vi "waveform temp.vi"() -> ()   [LabVIEW 2025]
panel:
  out "slide 2":u8(slide) scale=0.0..100.0
  out "slide 1":dbl(slide) scale=0.0..10.0
  out "iteration 2":dbl
  out "iteration 1":dbl
  out "Waveform Chart":dbl(graph)
  in  "mil per sec to wait":dbl
  in  "no of loops":dbl
  out "Waveform Graph":dbl[](graph)
  in  "mil per sec":dbl
  in  "no of loops":dbl
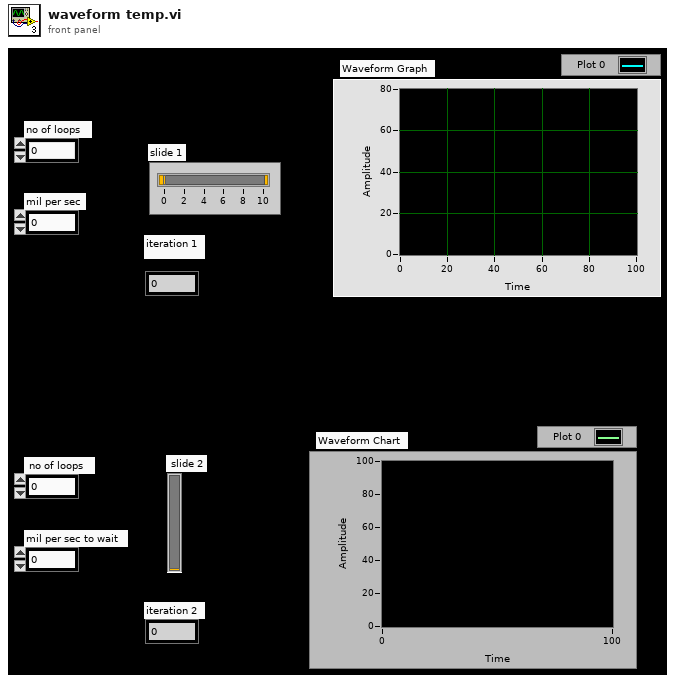
[diagram p1: front panel]
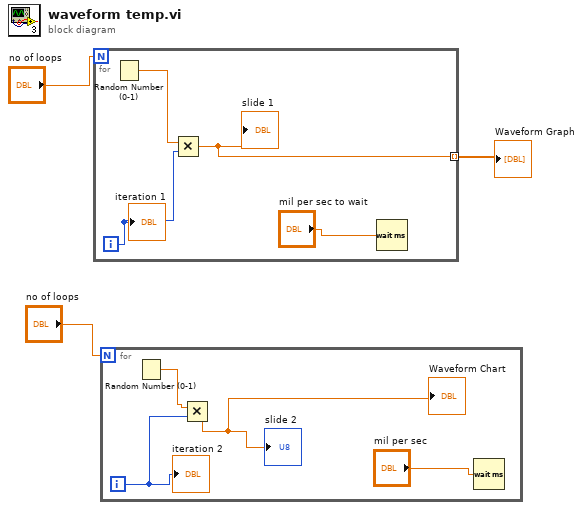
[diagram p0: block diagram]
diagram:
  n1 = for {
    N: "no of loops" -> [_]
    tunnel: [w4] -> w1 mode=indexing
    i -> [w6]
    n2 = Random Number (0-1)() -> (number: 0 to 1=w5:dbl)
    n3 = Multiply(x=w5, y=w6) -> (x*y=w4:dbl)
    "slide 1" <- w4
    n4 = Wait (ms)(milliseconds to wait="mil per sec to wait") -> ()  [unwired: 1 out]
    "iteration 1" <- w6
  }
  "Waveform Graph" <- w1
  n5 = for {
    N: "no of loops" -> [_]
    i -> [w9]
    n6 = Random Number (0-1)() -> (number: 0 to 1=w10:dbl)
    n7 = Multiply(x=w10, y=w9) -> (x*y=→"Waveform Chart" →"slide 2":dbl)
    n8 = Wait (ms)(milliseconds to wait="mil per sec") -> ()  [unwired: 1 out]
    "iteration 2" <- w9
  }
